vi "UI Interlocks.vi"(9 "Macro":cluster{"New":T1, "Saved":T1, "Name":string}, 11 "Refs":T5) -> ()   [LabVIEW 2023]
doc: "Enables and disables controls based on the current state of the interface."
uses:
  CTLs/Refs.ctl
  CTLs/Macro Cluster V3.ctl
  CTLs/Macro Config V3.ctl
  CTLs/Step V3.ctl
  CTLs/Step Type V3.ctl
  <userlib>/_MGI/Application Control/MGI Gray if/MGI Gray if False.vi
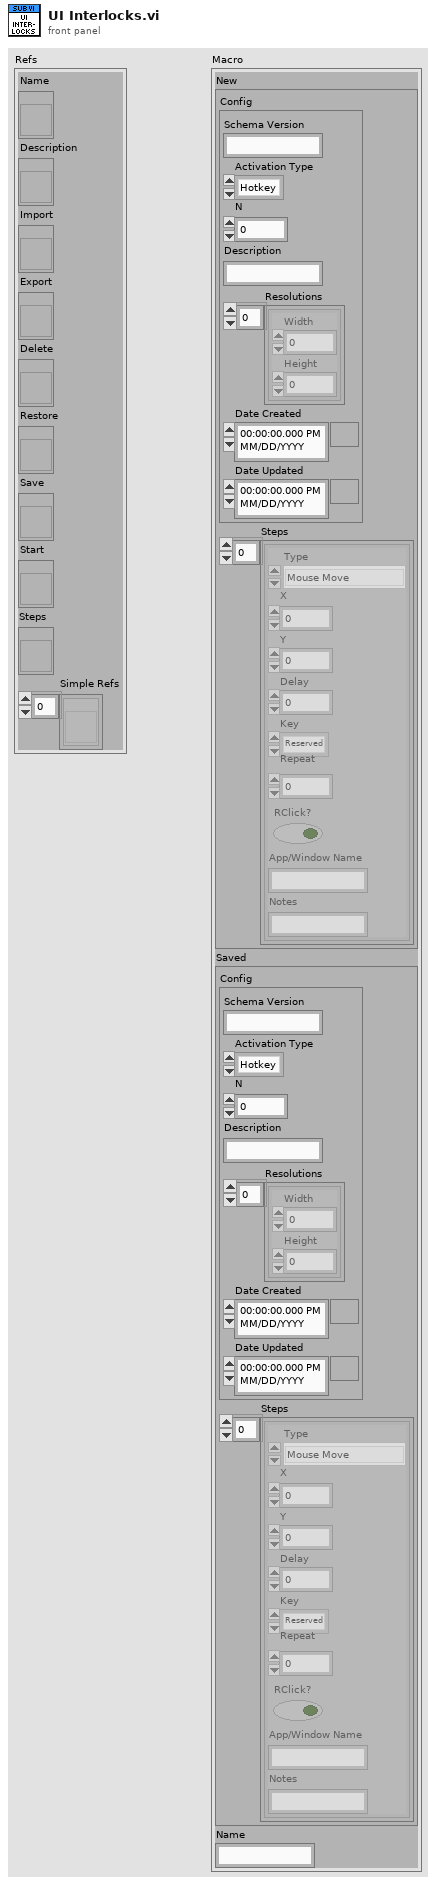
[diagram p1: front panel]
types:
  T1 = typedef "Macro Cluster V3.ctl" = cluster{"Config":T2, "Steps":T3[]}
  T2 = typedef "Macro Config V3.ctl" = cluster{"Schema Version":string, "Activation Type":enum32{"Hotkey", "Automatic"}, "N":i32, "Description":string, "Resolutions":cluster{"Width":i16, "Height":i16}[], "Date Created":timestamp, "Date Updated":timestamp}
  T3 = typedef "Step V3.ctl" = cluster{"Type":T4, "X":i32, "Y":i32, "Delay":i32, "Key":u8, "Repeat":i32, "RClick?":bool, "App/Window Name":string, "Notes":string}
  T4 = typedef "Step Type V3.ctl" = enum16{"Mouse Move", "Mouse Click", "Key Press", "Wait", "Mouse Down", "Mouse Up", "Key Down", "Key Up", "Run Application", "Maximize Window", "Restore Window", "Minimize Window", "Close Window", "Bring Window to Front", "Send Window to Back"}
  T5 = typedef "Refs.ctl" = cluster{"Name":refnum<vi>, "Description":refnum<vi>, "Import":refnum<vi>, "Export":refnum<vi>, "Delete":refnum<vi>, "Restore":refnum<vi>, "Save":refnum<vi>, "Start":refnum<vi>, "Steps":refnum<vi>, "Simple Refs":refnum<vi>[]}
  T6 = enum8{"Enabled", "Disabled", "Disabled and Grayed Out"}
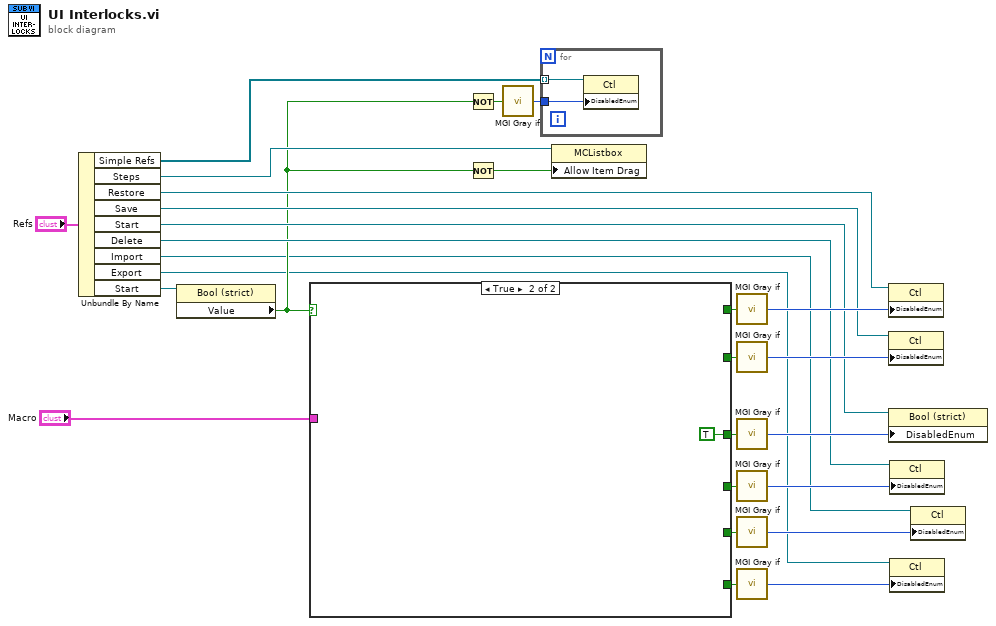
[diagram p0: block diagram]
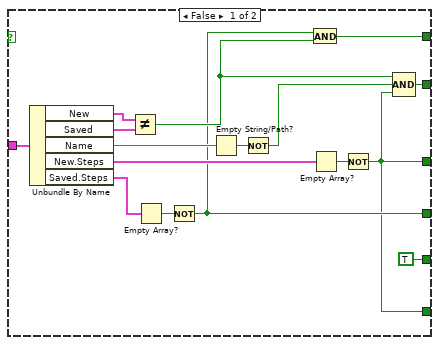
[diagram p2: hidden frame]
diagram:
  n1 = Unbundle By Name("Refs") -> ("Simple Refs"=w10:refnum<vi>[], "Steps"=w26:refnum<vi>, "Restore"=w13:refnum<vi>, "Save"=w14:refnum<vi>, "Start"=w15:refnum<vi>, "Delete"=w16:refnum<vi>, "Import"=w5:refnum<vi>, "Export"=w4:refnum<vi>, "Start"=w11:refnum<vi>)
  n2 = property class="Bool (strict)"(reference=w11) -> ("Value"=w7:bool)  [unwired: 1 in, 2 out]
  n3 = case shown="True" w7 {
    tunnel: [w40 _] -> w25
    tunnel: [w28 TRUE] -> w23
    tunnel: [w30 _] -> w20
    tunnel: [w31 _] -> w18
    tunnel: "Macro" -> [w33 _]
    tunnel: [TRUE _] -> w2
    tunnel: [w28 _] -> w1
    frame False {
      n4 = Unbundle By Name(w33) -> ("New"=w36:T1, "Saved"=w37:T1, "Name"=w39:string, "New.Steps"=w38:T3[], "Saved.Steps"=w34:T3[])
      n5 = Not Equal?(x=w36, y=w37) -> (x != y?=w32:bool)
      n6 = Empty Array?(array=w34) -> (empty?=w35:bool)
      n7 = Not(x=w35) -> (.not. x?=w31:bool)
      n8 = Empty String/Path?(string/path=w39) -> (empty?=w42:bool)
      n9 = Not(x=w42) -> (.not. x?=w41:bool)
      n10 = And(x=w31, y=w32) -> (x .and. y?=w30:bool)
      n11 = Empty Array?(array=w38) -> (empty?=w43:bool)
      n12 = Not(x=w43) -> (.not. x?=w28:bool)
      n13 = Compound Arithmetic op=AND(w32, w41, w28) -> (w40:bool)
    }
    frame True {
    }
  }
  n14 = Not(x=w7) -> (.not. x?=w8:bool)
  n15 = Not(x=w7) -> (.not. x?=w6:bool)
  n16 = call-poly <userlib>:"MGI Gray if.vi"("Boolean"=w8) -> ("Disabled"=w9:T6)
  n17 = for {
    tunnel: w10 -> [w46] mode=indexing
    tunnel: w9 -> [w45]
    n18 = property class="Ctl"(reference=w46, "DisabledEnum"=w45) -> ()  [unwired: 1 in, 2 out]
  }
  n19 = property class="MCListbox"(reference=w26, "Allow Item Drag"=w6) -> ()  [unwired: 1 in, 2 out]
  n20 = call-poly <userlib>:"MGI Gray if.vi"("Boolean"=w20) -> ("Disabled"=w21:T6)
  n21 = call-poly <userlib>:"MGI Gray if.vi"("Boolean"=w25) -> ("Disabled"=w24:T6)
  n22 = call-poly <userlib>:"MGI Gray if.vi"("Boolean"=w23) -> ("Disabled"=w22:T6)
  n23 = call-poly <userlib>:"MGI Gray if.vi"("Boolean"=w18) -> ("Disabled"=w19:T6)
  n24 = call-poly <userlib>:"MGI Gray if.vi"("Boolean"=w2) -> ("Disabled"=w27:T6)
  n25 = call-poly <userlib>:"MGI Gray if.vi"("Boolean"=w1) -> ("Disabled"=w3:T6)
  n26 = property on="Property Node" class="Ctl"(reference=w13, "DisabledEnum"=w21) -> ()  [unwired: 1 in, 2 out]
  n27 = property on="Property Node" class="Ctl"(reference=w14, "DisabledEnum"=w24) -> ()  [unwired: 1 in, 2 out]
  n28 = property on="Property Node" class="Bool (strict)"(reference=w15, "DisabledEnum"=w22) -> ()  [unwired: 1 in, 2 out]
  n29 = property on="Property Node" class="Ctl"(reference=w16, "DisabledEnum"=w19) -> ()  [unwired: 1 in, 2 out]
  n30 = property on="Property Node" class="Ctl"(reference=w4, "DisabledEnum"=w3) -> ()  [unwired: 1 in, 2 out]
  n31 = property on="Property Node" class="Ctl"(reference=w5, "DisabledEnum"=w27) -> ()  [unwired: 1 in, 2 out]
